vi "Deep Learning Object Detection.vi"() -> ()   [LabVIEW 2018]
doc: "Demonstrates the usage of \"IMAQ DL Model Detect Objects\" to perform Object Detection using Deep Learning for Defect Inspection application."
uses:
  <vilib>/vision/Deep Learning.llb/IMAQ DL Model Objects.ctl
  <vilib>/vision/Deep Learning.llb/IMAQ DL Model Type.ctl
  <vilib>/vision/Deep Learning.llb/IMAQ DL Model Detect Objects Node Names.ctl
  <vilib>/vision/Deep Learning.llb/IMAQ DL Model Label.ctl
  <vilib>/vision/NI_Vision_Development_Module.lvlib
panel:
  out "Detected Defects":T1[](array[typedef]) {"Bounding Box"."y" format="%.2f"; "Bounding Box"."x" format="%.2f"}
  in  "Stop":bool
  out "Inspection Image":T2(plugin-control)
  in  "Minimum Score Threshold":sgl=0.70000005 min=0 max=1 step=0.1 format="%.3g"
  in  "Select Image":i32(slide) min=0 max=6 step=1 scale=0.0..6.0
  # "Overview: Demonstrates the use of the Model Importer APIs to perform Object detection using Deep Learning.\nRequirements: LabVIEW Full Development System 64 bit, Vision Development Module 2018\nInstructions:\n1. Run the VI.\n2. Choose a specific Image using the Select Image slider control\n3. Observe the Bounding box values for the defects under Detected Defects\n4. Click Stop to stop the VI."
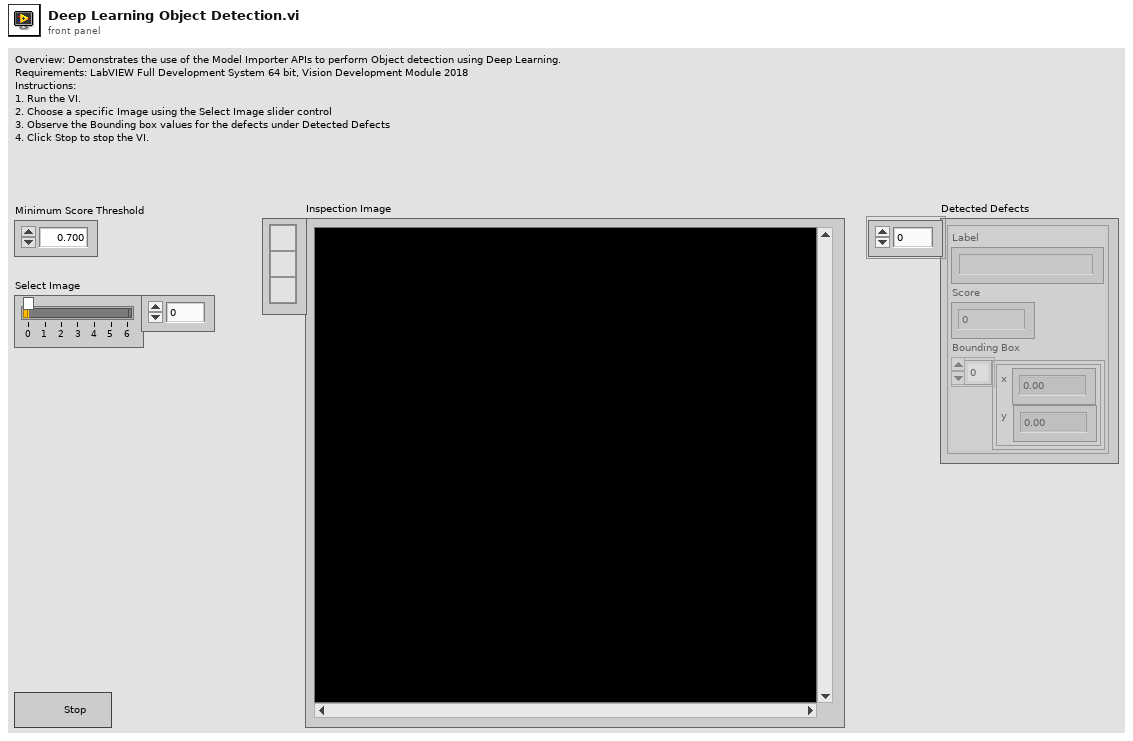
[diagram p1: front panel]
types:
  T1 = typedef "IMAQ DL Model Objects.ctl" = cluster{"Label":string, "Score":sgl, "Bounding Box":cluster{"x":sgl, "y":sgl}[]}
  T2 = typedef "IMAQ Image.ctl" = refnum<image>
  T3 = typedef "Image Type" = u32
  T4 = typedef "IMAQ DL Model Type.ctl" = i32
  T5 = typedef "IMAQ DL Model Refnum.ctl" = refnum<k20>
  T6 = typedef "IMAQ DL Model Label.ctl" = cluster{"ID":u32, "Label":string}
  T7 = typedef "IMAQ DL Model Detect Objects Node Names.ctl" = cluster{"Number of Objects":string, "Labels":string, "Scores":string, "Bounding Boxes":string}
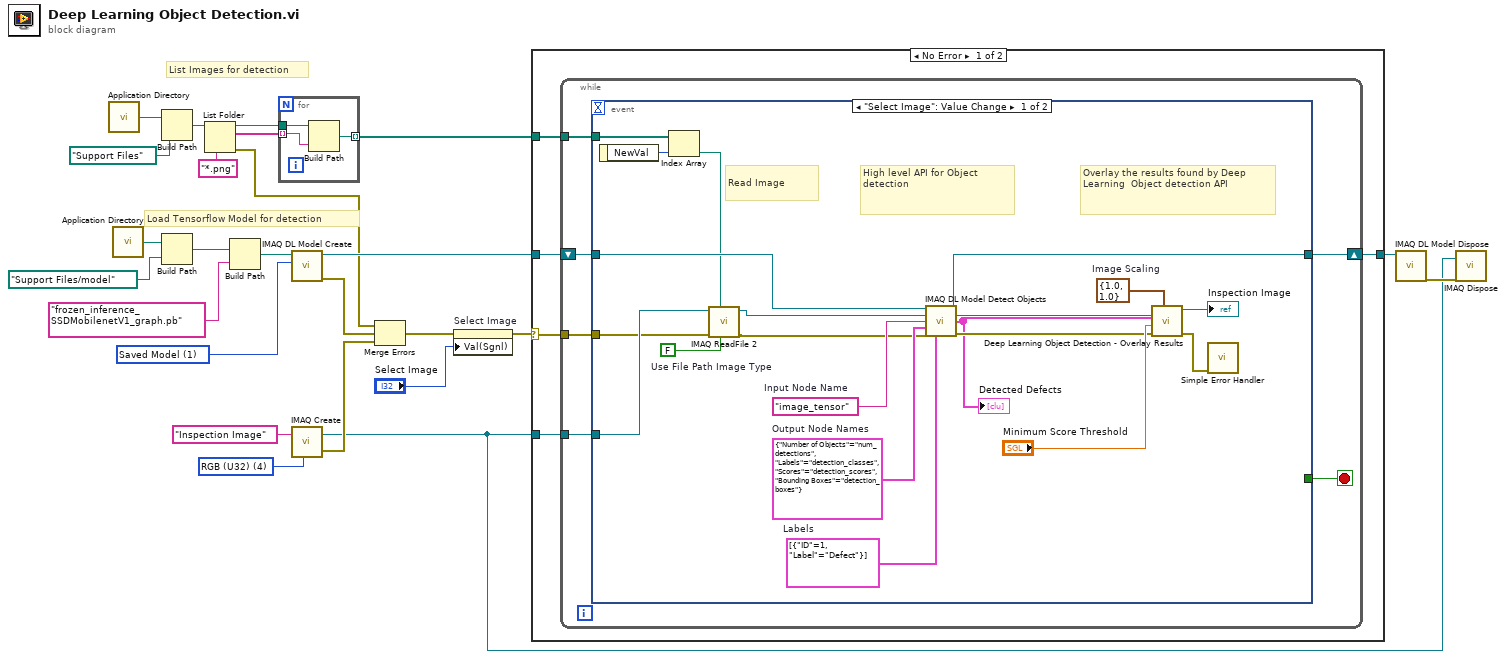
[diagram p0: block diagram]
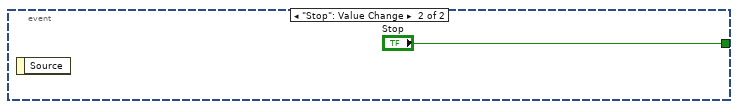
[diagram p2: hidden frame]
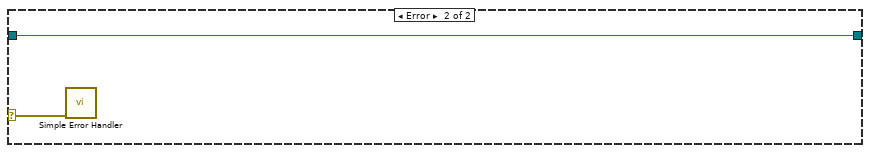
[diagram p3: hidden frame]
diagram:
  w6 = T3 4 items=["Grayscale (U8)", "Grayscale (I16)", "Grayscale (SGL)", "Complex (CSG)", "RGB (U32)", "HSL (U32)", "RGB (U64)", "Grayscale (U16)"] ("Image Type")
  w5 = T4 1 items=["Frozen Graph", "Saved Model"] ("Model Type")
  # "Load Tensorflow Model for detection"
  # "List Images for detection"
  n1 = call <vilib>:"Application Directory.vi"() -> ("Application Directory"=w2:path)
  n2 = call <vilib>:"Application Directory.vi"() -> ("Application Directory"=w1:path)
  n3 = Build Path(base path=w2, name or relative path=path "Support Files" ("path out")) -> (appended path=w21:path)
  n4 = Build Path(base path=w1, name or relative path=path "Support Files/model" ("path out")) -> (appended path=w14:path)
  n5 = List Folder(path=w21, pattern="*.png") -> (path out=w19:path, filenames=w18:string[], error out=w11:errorcluster)  [unwired: 1 in, 2 out]
  n6 = Build Path(base path=w14, name or relative path="frozen_inference_SSDMobilenetV1_graph.pb") -> (appended path=w25:path)
  n7 = for {
    tunnel: w19 -> [w28]
    tunnel: w18 -> [w27] mode=indexing
    tunnel: [w26] -> w17 mode=indexing
    n8 = Build Path(base path=w28, name or relative path=w27) -> (appended path=w26:path)
  }
  n9 = call-poly "IMAQ DL Model Create"("Model Type"=w5, "File Path"=w25) -> ("error out"=w13:errorcluster, "Model Refnum"=w24:T5)  [unwired: 8 in]
  n10 = call "IMAQ Create"("Image Name"="Inspection Image", "Image Type"=w6) -> ("New Image"=w3:T2, "error out"=w12:errorcluster)  [unwired: 3 in]
  n11 = Merge Errors(w11, w13, w12) -> (w8:errorcluster)
  n12 = property on="Select Image" class="Slide (strict)"(error in=w8, "Val(Sgnl)"="Select Image") -> (error out=w9:errorcluster)  [unwired: 1 in, 1 out]
  n13 = case shown="No Error" w9 {
    selector: w9 -> [w29 w61]
    tunnel: w24 -> [w33 w62]
    tunnel: [w32 w62] -> w23
    tunnel: w17 -> [w31 _]
    tunnel: w3 -> [w30 _]
    frame No Error {
      n14 = while {
        shift-right: [w37] -> w32
        shift-left: w33 -> [w39]
        tunnel: w31 -> [w36]
        tunnel: w30 -> [w35]
        tunnel: w29 -> [w34]
        stop <- w38 stop-if-true
        n15 = event shown="[0] \"Select Image\": Value Change" {
          selector: _ -> [_ _]
          dyn-events: _ -> [_ _]
          timeout: _ -> [_ _]
          tunnel: w39 -> [w59 _]
          tunnel: [_ "Stop"] -> w38
          tunnel: [w58 _] -> w37
          tunnel: w36 -> [w54 _]
          tunnel: w35 -> [w52 _]
          tunnel: w34 -> [w49 _]
          event "Select Image": Value Change {
            w42 = T6[] [{"ID"=1, "Label"="Defect"}]  # Labels
            w43 = FALSE  # Use File Path Image Type
            w47 = T7 {"Number of Objects"="num_detections", "Labels"="detection_classes", "Scores"="detection_scores", "Bounding Boxes"="detection_boxes"}  # Output Node Names
            w48 = "image_tensor"  # Input Node Name
            w51 = cluster{"X":dbl, "Y":dbl} {"X"=1.0, "Y"=1.0}  # Image Scaling
            # "Overlay the results found by Deep Learning  Object detection API"
            # "High level API for Object detection"
            # "Read Image"
            n16 = event-data() -> ("NewVal"=w45:i32)  [unwired: 1 in]
            n17 = Index Array(array=w54, index=w45) -> (element=w53:path)
            n18 = call "IMAQ ReadFile 2"("Use File Path Image Type"=w43, "File Path"=w53, "error in (no error)"=w49, "Image"=w52) -> ("error out"=w40:errorcluster, "Image Out"=w41:T2)  [unwired: 3 in, 3 out]
            n19 = call "IMAQ DL Model Detect Objects"("Model Refnum In"=w59, "Image"=w41, "Input Node Name"=w48, "Output Node Names"=w47, "error in (no error)"=w40, "Labels"=w42) -> ("Model Refnum Out"=w58:T5, "Image (duplicate)"=w50:T2, "Detected Objects"=w46:T1[], "error out"=w55:errorcluster)  [unwired: 5 in, 1 out]
            "Detected Defects" <- w46
            n20 = call "Deep Learning Object Detection - Overlay Results.vi"("Image Scaling"=w51, "error in (no error)"=w55, "Minimum Score Threshold"="Minimum Score Threshold", "Detected Objects"=w46, "Image In"=w50) -> ("error out"=w44:errorcluster, "Image Out"=→"Inspection Image":T2)  [unwired: 5 in]
            n21 = call <vilib>:"Simple Error Handler.vi"("error in (no error)"=w44) -> ()  [unwired: 4 in, 5 out]
          }
          event "Stop": Value Change {
            n22 = event-data() -> ()  [unwired: 1 in, 1 out]
          }
        }
      }
    }
    frame Error {
      n23 = call <vilib>:"Simple Error Handler.vi"("error in (no error)"=w61) -> ()  [unwired: 4 in, 5 out]
    }
  }
  n24 = call "IMAQ DL Model Dispose"("Model Refnum"=w23) -> ("error out"=w4:errorcluster)  [unwired: 10 in]
  n25 = call "IMAQ Dispose"("Image"=w3, "error in (no error)"=w4) -> ()  [unwired: 4 in, 1 out]
